vi "Configure Voltage Limit.vi"(0 "VISA resource name":refnum<visa-resource-name>, 5 "Address (0)":dbl min=0.0 max=31.0 step=1.0 format="%#.0p", 7 "Max Voltage Limit (80.000 V)":dbl=80.0 min=0.0 max=150.0 step=0.001 format="%.3f", 9 "Min Voltage Limit (0.000 V)":dbl min=0.0 max=150.0 step=0.001 format="%.3g", 11 "error in (no error)":errorcluster) -> (4 "VISA resource name out":refnum<visa-resource-name>, 15 "error out":errorcluster)   [LabVIEW 2020, in "BK Precision 911X Series.lvlib"]
doc: "Configures the maximum and minimum voltage limit."
uses:
  BK Precision 911X Series.lvlib
panel:
  # "V"
  # "V"
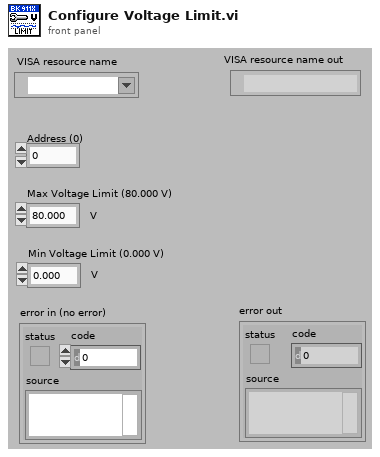
[diagram p1: front panel]
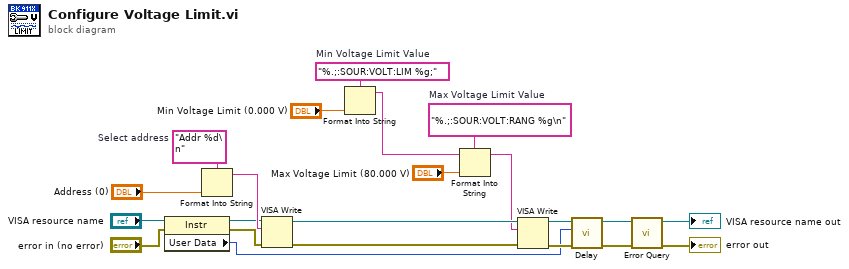
[diagram p0: block diagram]
diagram:
  w14 = "%.;:SOUR:VOLT:RANG %g\n"  # Max Voltage Limit Value
  w10 = "Addr %d\n"  # Select address
  w15 = "%.;:SOUR:VOLT:LIM %g;"  # Min Voltage Limit Value
  n1 = property class="Instr"(reference="VISA resource name", error in="error in (no error)") -> (reference out=w5:refnum<visa-resource-name>, error out=w2:errorcluster, "User Data"=w1:u32)
  n2 = Format Into String(format string=w10, "Address (0)") -> (resulting string=w20:string)  [unwired: 2 in, 1 out]
  n3 = VISA Write(VISA resource name=w5, write buffer=w20, error in (no error)=w2) -> (VISA resource name out=w17:refnum<visa-resource-name>, error out=w18:errorcluster)  [unwired: 1 out]
  n4 = Format Into String(format string=w15, "Min Voltage Limit (0.000 V)") -> (resulting string=w13:string)  [unwired: 2 in, 1 out]
  n5 = Format Into String(format string=w14, initial string=w13, "Max Voltage Limit (80.000 V)") -> (resulting string=w11:string)  [unwired: 1 in, 1 out]
  n6 = VISA Write(VISA resource name=w17, write buffer=w11, error in (no error)=w18) -> (VISA resource name out=w9:refnum<visa-resource-name>, error out=w8:errorcluster)  [unwired: 1 out]
  n7 = call "Delay.vi"("error in (no error)"=w8, "Delay Time (0 ms)"=w1, "VISA resource name"=w9) -> ("error out"=w6:errorcluster, "VISA resource name out"=w7:refnum<visa-resource-name>)  [unwired: 7 in]
  n8 = call "Error Query.vi"("error in (no error)"=w6, "VISA resource name"=w7) -> ("error out"=→"error out":errorcluster, "VISA resource name out"=→"VISA resource name out":refnum<visa-resource-name>)  [unwired: 6 in, 2 out]
